vi "Full Stoch State-Space.vi"(0 "kt":dbl=0.00064, 1 "kr":dbl=0.00064, 4 "m":dbl=0.0038, 6 "Jx":dbl=0.0038, 9 "ut":dbl=0.00064, 10 "Jy":dbl=0.0038, 12 "Jz":dbl=0.0071) -> (8 "Altitude Deterministic State-Space Model":T1 {"Transport Delay" format="%.2f"; "D" format="%#.2g"; "C" format="%#.2g"; "B" format="%#.2g"; "A" format="%#.2g"; "properties"."Sampling Time" format="%#.6p"; "properties"."Output Delays" format="%.4f"; "properties"."Input Delays" format="%.4f"}, 11 "Translational Deterministic State-Space Model":T1 {"Transport Delay" format="%.2f"; "D" format="%#.2g"; "C" format="%#.2g"; "B" format="%#.2g"; "A" format="%#.2g"; "properties"."Sampling Time" format="%#.6p"; "properties"."Output Delays" format="%.4f"; "properties"."Input Delays" format="%.4f"}, 13 "Angular Stochastic State-Space Model":T3 {"H" format="%#.2g"; "D" format="%#.2g"; "C" format="%#.2g"; "A" format="%#.2g"; "B" format="%#.2g"; "G" format="%#.2g"; "Sampling Time (s)" format="%.2f"}, 14 "Equation":picture, 15 "Equation 3":picture, 16 "Angular Deterministic State-Space Model":T1 {"Transport Delay" format="%.2f"; "D" format="%#.2g"; "C" format="%#.2g"; "B" format="%#.2g"; "A" format="%#.2g"; "properties"."Sampling Time" format="%#.6p"; "properties"."Output Delays" format="%.4f"; "properties"."Input Delays" format="%.4f"}, 17 "Equation 2":picture, 18 "Translational Stochastic State-Space Model":T3 {"H" format="%#.2g"; "D" format="%#.2g"; "C" format="%#.2g"; "A" format="%#.2g"; "B" format="%#.2g"; "G" format="%#.2g"; "Sampling Time (s)" format="%.2f"}, 19 "Altitude Stochastic State-Space Model":T3 {"H" format="%#.2g"; "D" format="%#.2g"; "C" format="%#.2g"; "A" format="%#.2g"; "B" format="%#.2g"; "G" format="%#.2g"; "Sampling Time (s)" format="%.2f"})   [LabVIEW 2017]
uses:
  <vilib>/addons/Control Design/_Stochastic Systems/Stochastic Systems.llb/Stochastic Systems SubVIs/cd_Stochastic State-Space Model.ctl
  <vilib>/addons/Control Design/_Model Construction/Model Typedefs.llb/CD State Space Model (MIMO).ctl
  <vilib>/addons/Control Design/_Model Construction/Model Typedefs.llb/CD General Elements.ctl
  <vilib>/Analysis/7linalg.llb/Create Special Real Matrix.vi
  <vilib>/addons/Control Design/_Stochastic Systems/Stochastic Systems.llb/CD Construct Stochastic Model (Numeric).vi
  <vilib>/addons/Control Design/_Stochastic Systems/NI_CD_Stochastic Systems.lvlib
  <vilib>/Analysis/NI_AALPro.lvlib
  <vilib>/addons/Control Design/_Utility/NI_CD_Model Viewer.lvlib
  <vilib>/addons/Control Design/_State-Space Analysis/NI_CD_State-Space Analysis.lvlib
  <vilib>/addons/Control Design/_Model Construction/NI_LinSys_Model Typedefs.lvlib
panel:
  out "Observability  Matrix 3":dbl[][](array[numeric]) format="%#.2g"
  out "Is Observable 3":bool
  out "Controllability Matrix 3":dbl[][](array[numeric])=[[1.0, 0.0, 6.0], [0.0, 1.0, -1.0], [0.0, 0.0, 0.0]] format="%.2f"
  out "Is Controllable 3":bool
  out "Observability  Matrix 2":dbl[][](array[numeric]) format="%#.2g"
  out "Is Observable 2":bool
  out "Controllability Matrix 2":dbl[][](array[numeric])=[[1.0, 0.0, 6.0], [0.0, 1.0, -1.0], [0.0, 0.0, 0.0]] format="%.2f"
  out "Is Controllable 2":bool
  out "Observability  Matrix":dbl[][](array[numeric]) format="%#.2g"
  out "Is Observable":bool
  out "Controllability Matrix":dbl[][](array[numeric])=[[1.0, 0.0, 6.0], [0.0, 1.0, -1.0], [0.0, 0.0, 0.0]] format="%.2f"
  out "Is Controllable":bool
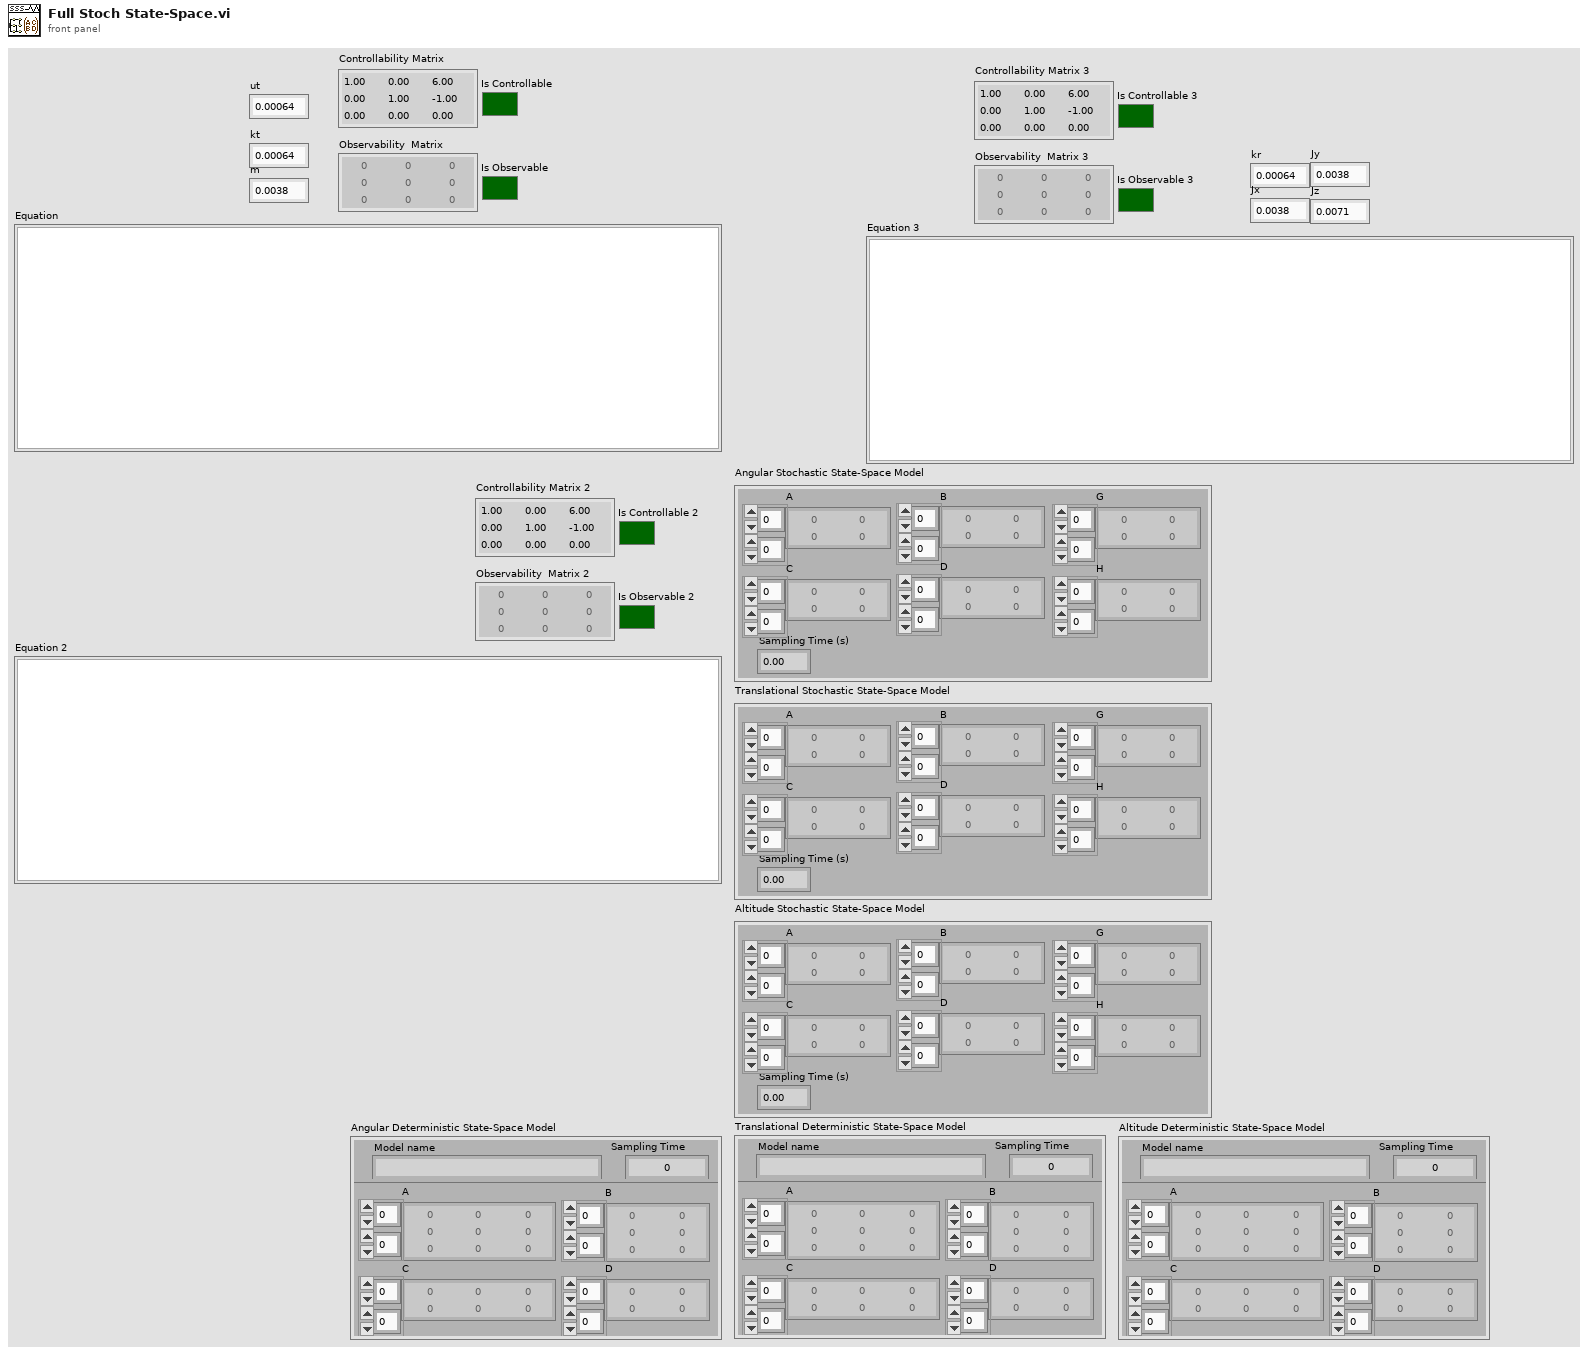
[diagram p1: front panel]
types:
  T1 = typedef "NI_LinSys_Model Typedefs.lvlib/CD State Space Model (MIMO).ctl" = cluster{"properties":T2, "A":dbl[][], "B":dbl[][], "C":dbl[][], "D":dbl[][], "StateNames":string[], "Transport Delay":dbl[][]}
  T2 = typedef "NI_LinSys_Model Typedefs.lvlib/CD General Elements.ctl" = cluster{"Model name":string, "Input names":string[], "Output names":string[], "Input Delays":dbl[], "Output Delays":dbl[], "Sampling Time":dbl, "Notes":string}
  T3 = typedef "NI_CD_Stochastic Systems.lvlib/cd_Stochastic State-Space Model.ctl" = cluster{"Sampling Time (s)":dbl, "G":dbl[][], "B":dbl[][], "A":dbl[][], "C":dbl[][], "D":dbl[][], "H":dbl[][]}
  T4 = typedef "NI_Matrix.lvlib/RealMatrix.ctl" = dbl[][]
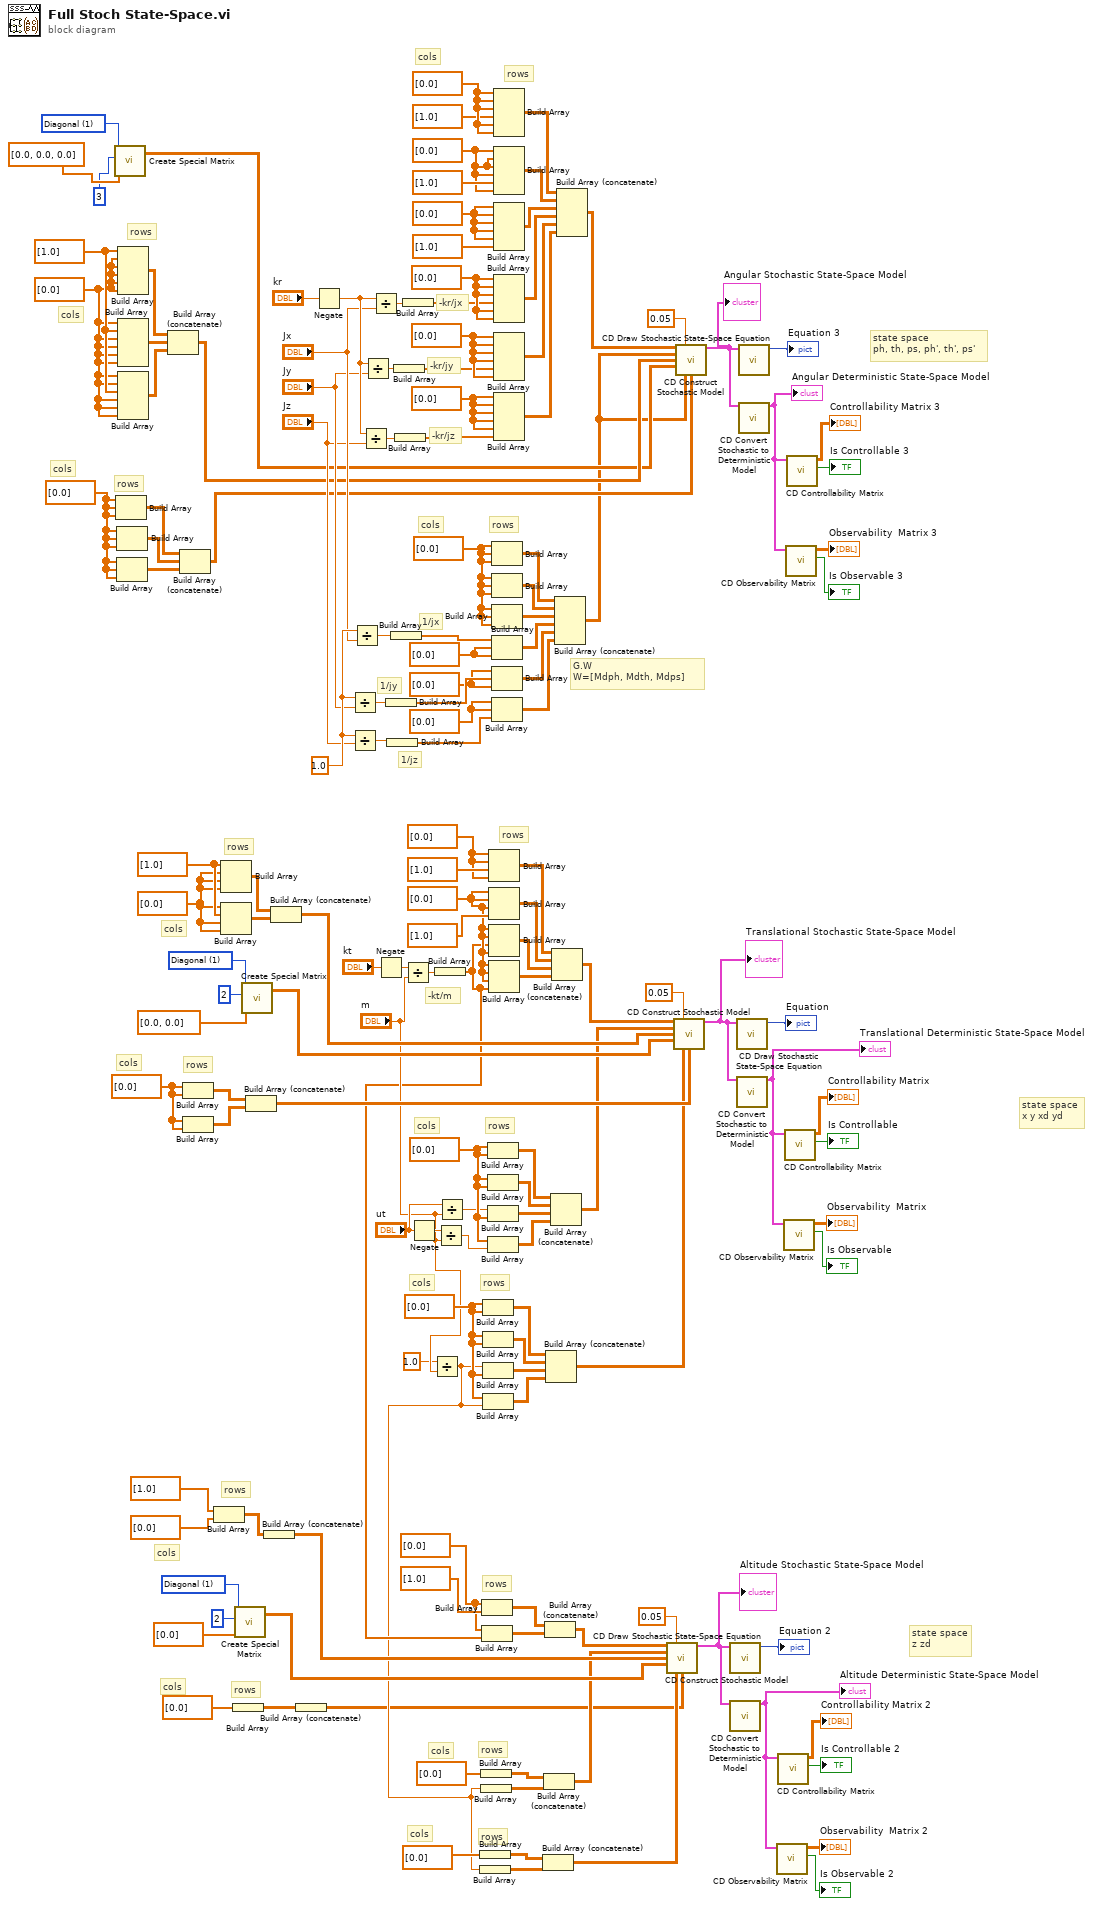
[diagram p0: block diagram]
diagram:
  w1 = dbl[] [0.0] ("element")
  w20 = dbl[] [1.0] ("element")
  w19 = dbl[] [0.0] ("element")
  w27 = 1 items=["Identity", "Diagonal", "Toepliz", "Vandermonde", "Companion", "Hankel", "Hadamard", "Wilkinson", "Hilbert", "Inverse Hilbert", "Rosser", "Pascal"] ("matrix type")
  w31 = 1.0 ("x")
  w35 = dbl[] [0.0] ("element")
  w36 = dbl[] [0.0] ("element")
  w37 = dbl[] [0.0] ("element")
  w21 = dbl[] [0.0] ("element")
  w60 = dbl[] [0.0] ("element")
  w59 = dbl[] [0.0] ("element")
  w58 = dbl[] [0.0] ("element")
  w64 = dbl[] [0.0] ("element")
  w2 = dbl[] [0.0] ("element")
  w68 = dbl[] [0.0] ("element")
  w99 = 1 items=["Identity", "Diagonal", "Toepliz", "Vandermonde", "Companion", "Hankel", "Hadamard", "Wilkinson", "Hilbert", "Inverse Hilbert", "Rosser", "Pascal"] ("matrix type")
  w81 = dbl[] [0.0] ("element")
  w110 = dbl[] [0.0] ("element")
  w136 = dbl[] [0.0] ("element")
  w106 = dbl[] [1.0] ("element")
  w105 = dbl[] [0.0] ("element")
  w142 = 1 items=["Identity", "Diagonal", "Toepliz", "Vandermonde", "Companion", "Hankel", "Hadamard", "Wilkinson", "Hilbert", "Inverse Hilbert", "Rosser", "Pascal"] ("matrix type")
  w119 = dbl[] [0.0] ("element")
  w103 = dbl[] [0.0] ("element")
  w121 = dbl[] [0.0] ("element")
  # "state space\nph, th, ps, ph', th', ps'"
  # "G.W\nW=[Mdph, Mdth, Mdps]"
  # "rows"
  # "cols"
  # "rows"
  # "cols"
  # "1/jz"
  # "1/jy"
  # "1/jx"
  # "rows"
  # "cols"
  # "-kr/jz"
  # "-kr/jy"
  # "-kr/jx"
  # "rows"
  # "cols"
  # "state space\nz zd"
  # "state space \nx y xd yd"
  # "rows"
  # "cols"
  # "rows"
  # "cols"
  # "rows"
  # "cols"
  # "rows"
  # "cols"
  # "rows"
  # "rows"
  # "cols"
  # "rows"
  # "cols"
  # "rows"
  # "cols"
  # "rows"
  # "cols"
  # "-kt/m"
  # "rows"
  n1 = call-poly <vilib>:"Create Special Matrix.vi"("matrix type"=w27, "matrix size"=3, "Input Vector1"=dbl[] [0.0, 0.0, 0.0]) -> ("Special Matrix"=w13:T4)  [unwired: 2 in, 1 out]
  n2 = Build Array(w1, w1, w1) -> (w18:T4)
  n3 = Build Array(w1, w1, w1) -> (w17:T4)
  n4 = Build Array(w1, w1, w1) -> (w16:T4)
  n5 = Build Array(w20, w19, w19, w19, w19, w19) -> (w22:T4)
  n6 = Build Array(w19, w20, w19, w19, w19, w19) -> (w23:T4)
  n7 = Build Array(w19, w19, w20, w19, w19, w19) -> (w24:T4)
  n8 = Build Array (concatenate)(w22, w23, w24) -> (w14:T4)
  n9 = Build Array (concatenate)(w18, w17, w16) -> (w10:T4)
  n10 = Build Array(w136, w136) -> (w138:T4)
  n11 = Build Array(w136, w136) -> (w137:T4)
  n12 = Build Array(dbl[] [1.0] ("element"), dbl[] [0.0] ("element")) -> (w97:T4)
  n13 = Build Array(w106, w105, w105, w105) -> (w139:T4)
  n14 = Build Array(w105, w106, w105, w105) -> (w140:T4)
  n15 = Build Array(dbl[] [0.0] ("element")) -> (w71:T4)
  n16 = call-poly <vilib>:"Create Special Matrix.vi"("matrix type"=w99, "matrix size"=2, "Input Vector1"=dbl[] [0.0]) -> ("Special Matrix"=w94:T4)  [unwired: 2 in, 1 out]
  n17 = call-poly <vilib>:"Create Special Matrix.vi"("matrix type"=w142, "matrix size"=2, "Input Vector1"=dbl[] [0.0, 0.0]) -> ("Special Matrix"=w133:T4)  [unwired: 2 in, 1 out]
  n18 = Build Array (concatenate)(w138, w137) -> (w130:T4)
  n19 = Build Array (concatenate)(w97) -> (w95:T4)
  n20 = Build Array (concatenate)(w139, w140) -> (w134:T4)
  n21 = Build Array (concatenate)(w71) -> (w70:T4)
  n22 = Negate(x="kr") -> (-x=w53:dbl)
  n23 = Divide(x=w31, y="Jy") -> (x/y=w44:dbl)
  n24 = Divide(x=w31, y="Jz") -> (x/y=w43:dbl)
  n25 = Divide(x=w31, y="Jx") -> (x/y=w41:dbl)
  n26 = Divide(x=w53, y="Jz") -> (x/y=w50:dbl)
  n27 = Divide(x=w53, y="Jy") -> (x/y=w49:dbl)
  n28 = Divide(x=w53, y="Jx") -> (x/y=w52:dbl)
  n29 = Negate(x="kt") -> (-x=w148:dbl)
  n30 = Build Array(w44) -> (w45:dbl[])
  n31 = Build Array(w43) -> (w46:dbl[])
  n32 = Build Array(w41) -> (w42:dbl[])
  n33 = Build Array(w49) -> (w48:dbl[])
  n34 = Build Array(w50) -> (w47:dbl[])
  n35 = Build Array(w52) -> (w51:dbl[])
  n36 = Divide(x=w148, y="m") -> (x/y=w147:dbl)
  n37 = Negate(x="ut") -> (-x=w118:dbl)
  n38 = Divide(x=1.0, y="m") -> (x/y=w72:dbl)
  n39 = Build Array(w147) -> (w80:dbl[])
  n40 = Divide(x=w118, y="m") -> (x/y=w117:dbl)
  n41 = Divide(x="ut", y="m") -> (x/y=w116:dbl)
  n42 = Build Array(dbl[] [0.0] ("element")) -> (w76:T4)
  n43 = Build Array(w72) -> (w75:T4)
  n44 = Build Array(dbl[] [0.0] ("element")) -> (w100:T4)
  n45 = Build Array(w72) -> (w77:T4)
  n46 = Build Array(w81, dbl[] [1.0] ("element")) -> (w101:T4)
  n47 = Build Array(w81, w80) -> (w102:T4)
  n48 = Build Array(w110, w110) -> (w113:T4)
  n49 = Build Array(w110, w110) -> (w112:T4)
  n50 = Build Array(w72, w110) -> (w111:T4)
  n51 = Build Array(w110, w72) -> (w114:T4)
  n52 = Build Array(w119, w119) -> (w145:T4)
  n53 = Build Array(w119, w119) -> (w144:T4)
  n54 = Build Array(w116, w119) -> (w143:T4)
  n55 = Build Array(w119, w117) -> (w146:T4)
  n56 = Build Array(w121, w121, dbl[] [1.0] ("element"), w121) -> (w151:T4)
  n57 = Build Array(w103, w103, w103, dbl[] [1.0] ("element")) -> (w152:T4)
  n58 = Build Array(w103, w103, w80, w103) -> (w153:T4)
  n59 = Build Array(w103, w103, w103, w80) -> (w150:T4)
  n60 = Build Array(w21, w21, w21) -> (w34:T4)
  n61 = Build Array(w21, w21, w21) -> (w33:T4)
  n62 = Build Array(w21, w21, w21) -> (w32:T4)
  n63 = Build Array(w42, w37, w37) -> (w38:T4)
  n64 = Build Array(w36, w45, w36) -> (w39:T4)
  n65 = Build Array(w35, w35, w46) -> (w40:T4)
  n66 = Build Array(w68, w68, w68, dbl[] [1.0] ("element"), w68, w68) -> (w61:T4)
  n67 = Build Array(w2, w2, w2, w2, dbl[] [1.0] ("element"), w2) -> (w62:T4)
  n68 = Build Array(w64, w64, w64, w64, w64, dbl[] [1.0] ("element")) -> (w63:T4)
  n69 = Build Array(w58, w58, w58, w51, w58, w58) -> (w57:T4)
  n70 = Build Array(w59, w59, w59, w59, w48, w59) -> (w56:T4)
  n71 = Build Array(w60, w60, w60, w60, w60, w47) -> (w55:T4)
  n72 = Build Array (concatenate)(w76, w75) -> (w74:T4)
  n73 = Build Array (concatenate)(w100, w77) -> (w91:T4)
  n74 = Build Array (concatenate)(w101, w102) -> (w96:T4)
  n75 = Build Array (concatenate)(w113, w112, w111, w114) -> (w107:T4)
  n76 = Build Array (concatenate)(w145, w144, w143, w146) -> (w129:T4)
  n77 = Build Array (concatenate)(w151, w152, w153, w150) -> (w135:T4)
  n78 = Build Array (concatenate)(w34, w33, w32, w38, w39, w40) -> (w9:T4)
  n79 = Build Array (concatenate)(w61, w62, w63, w57, w56, w55) -> (w15:T4)
  n80 = call-poly <vilib>:"CD Construct Stochastic Model.vi"("A"=w96, "Sampling Time (s)"=0.05, "B"=w91, "C"=w95, "D"=w94, "G"=w74, "H"=w70) -> ("Stochastic State-Space Model"=w89:T3)  [unwired: 7 in, 1 out]
  "Altitude Stochastic State-Space Model" <- w89
  n81 = call-poly <vilib>:"CD Construct Stochastic Model.vi"("A"=w135, "Sampling Time (s)"=0.05, "B"=w129, "C"=w134, "D"=w133, "G"=w107, "H"=w130) -> ("Stochastic State-Space Model"=w127:T3)  [unwired: 7 in, 1 out]
  "Translational Stochastic State-Space Model" <- w127
  n82 = call-poly <vilib>:"CD Construct Stochastic Model.vi"("A"=w15, "Sampling Time (s)"=0.05, "B"=w9, "C"=w14, "D"=w13, "G"=w9, "H"=w10) -> ("Stochastic State-Space Model"=w7:T3)  [unwired: 7 in, 1 out]
  "Angular Stochastic State-Space Model" <- w7
  n83 = call <vilib>:"CD Draw Stochastic State-Space Equation.vi"("Stochastic State-Space Model"=w89) -> ("Equation"=→"Equation 2":picture)  [unwired: 8 in, 2 out]
  n84 = call <vilib>:"CD Convert Stochastic to Deterministic Model.vi"("Stochastic State-Space Model"=w89) -> ("Deterministic State-Space Model"=w87:T1)  [unwired: 13 in, 1 out]
  "Altitude Deterministic State-Space Model" <- w87
  n85 = call <vilib>:"CD Draw Stochastic State-Space Equation.vi"("Stochastic State-Space Model"=w127) -> ("Equation"=→"Equation":picture)  [unwired: 8 in, 2 out]
  n86 = call <vilib>:"CD Convert Stochastic to Deterministic Model.vi"("Stochastic State-Space Model"=w127) -> ("Deterministic State-Space Model"=w125:T1)  [unwired: 13 in, 1 out]
  "Translational Deterministic State-Space Model" <- w125
  n87 = call <vilib>:"CD Draw Stochastic State-Space Equation.vi"("Stochastic State-Space Model"=w7) -> ("Equation"=→"Equation 3":picture)  [unwired: 8 in, 2 out]
  n88 = call <vilib>:"CD Convert Stochastic to Deterministic Model.vi"("Stochastic State-Space Model"=w7) -> ("Deterministic State-Space Model"=w5:T1)  [unwired: 13 in, 1 out]
  "Angular Deterministic State-Space Model" <- w5
  n89 = call <vilib>:"CD Observability Matrix.vi"("State-Space Model"=w87) -> ("Is Observable?"=→"Is Observable 2":bool, "Observability  Matrix"=→"Observability  Matrix 2":dbl[][])  [unwired: 7 in, 2 out]
  n90 = call <vilib>:"CD Controllability Matrix.vi"("State-Space Model"=w87) -> ("Is Controllable?"=→"Is Controllable 2":bool, "Controllability Matrix"=→"Controllability Matrix 2":dbl[][])  [unwired: 7 in, 2 out]
  n91 = call <vilib>:"CD Observability Matrix.vi"("State-Space Model"=w125) -> ("Is Observable?"=→"Is Observable":bool, "Observability  Matrix"=→"Observability  Matrix":dbl[][])  [unwired: 7 in, 2 out]
  n92 = call <vilib>:"CD Controllability Matrix.vi"("State-Space Model"=w125) -> ("Is Controllable?"=→"Is Controllable":bool, "Controllability Matrix"=→"Controllability Matrix":dbl[][])  [unwired: 7 in, 2 out]
  n93 = call <vilib>:"CD Observability Matrix.vi"("State-Space Model"=w5) -> ("Is Observable?"=→"Is Observable 3":bool, "Observability  Matrix"=→"Observability  Matrix 3":dbl[][])  [unwired: 7 in, 2 out]
  n94 = call <vilib>:"CD Controllability Matrix.vi"("State-Space Model"=w5) -> ("Is Controllable?"=→"Is Controllable 3":bool, "Controllability Matrix"=→"Controllability Matrix 3":dbl[][])  [unwired: 7 in, 2 out]
